vi "Sin Sum.vi"(11 "x":dbl) -> (3 "sin sum(x)":dbl)   [LabVIEW 2018]
doc: "Function creates the sin sum\nf(x) = 4/Pi * (sin(x)+sin(3x)/3 + sin(5x)/5) for input values x."
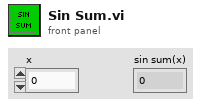
[diagram p1: front panel]
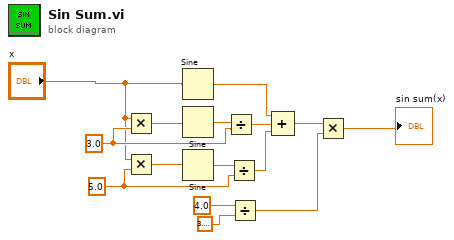
[diagram p0: block diagram]
diagram:
  w10 = 5.0 ("y")
  w12 = 3.0 ("y")
  n1 = Multiply(x="x", y=w12) -> (x*y=w14:dbl)
  n2 = Multiply(x="x", y=w10) -> (x*y=w15:dbl)
  n3 = Sine(x="x") -> (sin(x)=w9:dbl)
  n4 = Sine(x=w14) -> (sin(x)=w13:dbl)
  n5 = Sine(x=w15) -> (sin(x)=w11:dbl)
  n6 = Divide(x=w13, y=w12) -> (x/y=w8:dbl)
  n7 = Divide(x=w11, y=w10) -> (x/y=w7:dbl)
  n8 = Divide(x=4.0, y=3.141592653589793) -> (x/y=w3:dbl)
  n9 = Compound Arithmetic op=ADD(w9, w8, w7) -> (w6:dbl)
  n10 = Multiply(x=w6, y=w3) -> (x*y=→"sin sum(x)":dbl)
